vi "J1939 Host Automation API_Example.vi"() -> ()   [LabVIEW 2011]
uses:
  J1939 Host Automation API.lvlibp/APIs/Host Automation API/Controls/J1939_Verify DTC_Status.ctl
  J1939 Host Automation API.lvlibp/APIs/Host Automation API/Controls/J1939_DTC_Action.ctl
  J1939 Host Automation API.lvlibp
panel:
  out "error out":errorcluster
  out "Found DTCs":i32=6
  out "Status":T1
  in  "Expected DTC":string="75301.07"
  in  "Address":string="249"
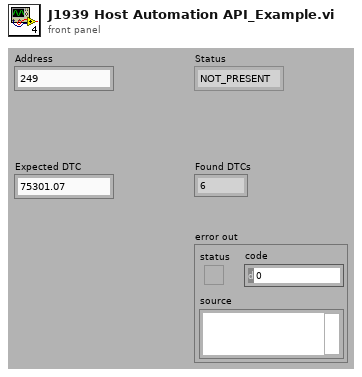
[diagram p1: front panel]
types:
  T1 = typedef "J1939 Host Automation API.lvlibp/J1939_Verify DTC_Status.ctl" = enum16{"NOT_PRESENT", "ACTIVE", "INACTIVE"}
  T2 = typedef "J1939 Host Automation API.lvlibp/J1939_DTC_Action.ctl" = enum16{"ALL", "ACTIVE", "INACTIVE"}
  T3 = typedef "J1939 Host Automation API.lvlibp/J1939 Custom Device.lvlib/J1939_stm_TCP Connection Info.ctl" = cluster{"connection ID":refnum<k5>, "Meta data":T4[]}
  T4 = typedef "J1939 Host Automation API.lvlibp/J1939 Custom Device.lvlib/J1939_stm_MetaDataElement.ctl" = string
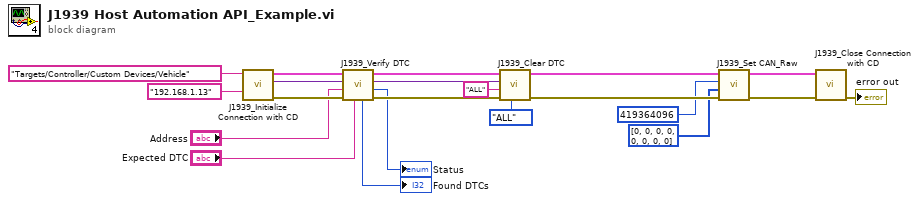
[diagram p0: block diagram]
diagram:
  n1 = call "J1939_Initialize Connection with CD.vi"("Unit Computer Address"="192.168.1.13", "Custom Device Path"="Targets/Controller/Custom Devices/Vehicle") -> ("error out"=w17:errorcluster, "Address Lookup Table"=w16:variant, "Connection Info"=w21:T3)  [unwired: 7 in]
  n2 = call "J1939_Verify DTC.vi"("Expected DTC"="Expected DTC", "error in"=w17, "Address"="Address", "Address Lookup Table"=w16, "Connection Info"=w21) -> ("error out"=w19:errorcluster, "Status"=→"Status":T1, "Address Lookup Table Out"=w18:variant, "Connection Info"=w20:T3, "Found DTCs"=→"Found DTCs":i32)  [unwired: 2 in]
  n3 = call "J1939_Clear DTC.vi"("Action"=J1939_DTC_Action."ALL", "error in"=w19, "Address (ALL)"="ALL" ("TLA (ALL)"), "Address Lookup Table"=w18, "Connection Info"=w20) -> ("error out"=w6:errorcluster, "Connection Info"=w8:T3)  [unwired: 4 in, 1 out]
  n4 = call "J1939_Set CAN_Raw.vi"("error in (no error)"=w6, "Data"=u8[] [0, 0, 0, 0, 0, 0, 0, 0], "Identifier"=u32 419364096, "Connection Info"=w8) -> ("error out"=w5:errorcluster, "Connection Info"=w7:T3)  [unwired: 6 in]
  n5 = call "J1939_Close Connection with CD.vi"("error in (no error)"=w5, "Connection Info"=w7) -> ("error out"=→"error out":errorcluster)  [unwired: 9 in]
